vi "Maximum Interval.vi"() -> (0 "New Acquisition Time":u32)   [LabVIEW 2021, in "Interval Timer.lvlib"]
uses:
  Interval Timer.lvlib
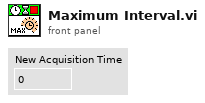
[diagram p1: front panel]
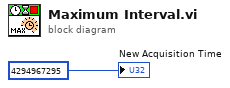
[diagram p0: block diagram]
diagram:
  "New Acquisition Time" <- u32 4294967295 ("New Acquisition Time")
